vi "03_data.vi"   [LabVIEW 2018]
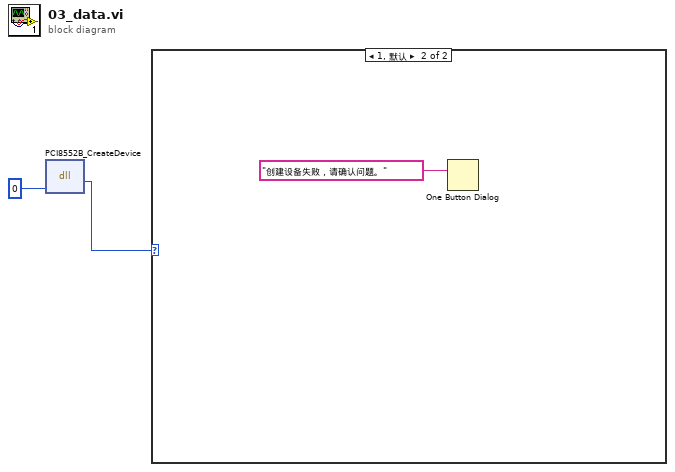
[diagram p0: block diagram]
diagram:
  n1 = dll-call lib="PCI8552B_32" fn="PCI8552B_CreateDevice" label="CreateDevice"("DeviceLgcID"=0) -> ("返回类型"=w1:i32)  [unwired: 4 in, 2 out]
  n2 = case shown="1, 默认" w1 {
    frame -1 {
    }
    frame 1, Default {
      n3 = One Button Dialog(message="创建设备失败，请确认问题。") -> ()  [unwired: 1 in, 1 out]
    }
  }
